vi "Test - Moving Objects Target.vi"() -> ()   [LabVIEW 2023]
doc: "This VI is used by the Moving Objects examples for VI Scripting."
panel:
  in  "Destination Cluster":cluster{}
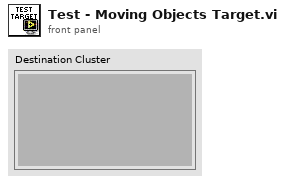
[diagram p1: front panel]
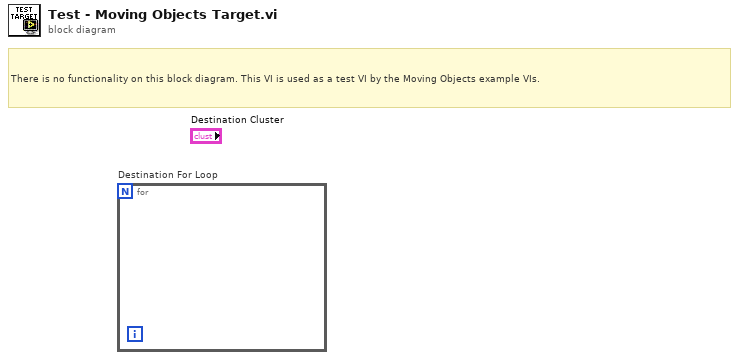
[diagram p0: block diagram]
diagram:
  # "There is no functionality on this block diagram. This VI is used as a test VI by the Moving Objects example VIs."
  n1 = for "Destination For Loop" {
  }
